vi "Hang Controller.vi"(8 "error in":errorcluster) -> ()   [LabVIEW 2019]
doc: "This VI executes continuously carrying out the current operation and responding to updates or new operations. It will often contain the timing or control code that is difficult to place directly in TeleOp. This VI generally opens all sensors and motors and isolates the rest of the robot code from knowing how the operations are carried out."
uses:
  <vilib>/Rock Robotics/WPI/Framework/Completion Status.ctl
  Hang Setpoints.ctl
  Hang Operations.ctl
  <vilib>/Rock Robotics/WPI/Solenoid/WPI_SolenoidValue.ctl
  <vilib>/Rock Robotics/WPI/Solenoid/WPI_SolenoidChannel.ctl
  <vilib>/Rock Robotics/WPI/ThirdParty/Phoenix-LabVIEW/Motor Controller/Controls/CTRE_Phoenix_MotorControl_ControlMode.ctl
  <vilib>/Rock Robotics/WPI/Solenoid/WPI_SolenoidOpenDouble.vi
  <vilib>/Rock Robotics/WPI/Solenoid/WPI_SolenoidSetEnum.vi
panel:
  in  "Interactive Values":T1
  out "Current\nCmd":string
  in  "Buttons":cluster{"Execute Cmd":bool, "Abort Cmd":bool}
  out "Command Timing":cluster{"Start Time (ms)":u32, "Iterations":i32}
  out "Status":T4
  # "Tip: It may be helpful to observe inputs and sensor values.\nYou may also want to display tuning or debugging controls."
  # "Interactive Command: You may fill in the settings for a command\nand schedule it with the Execute button. You can observe and abort\nany command while fine tuning the code for the controller."
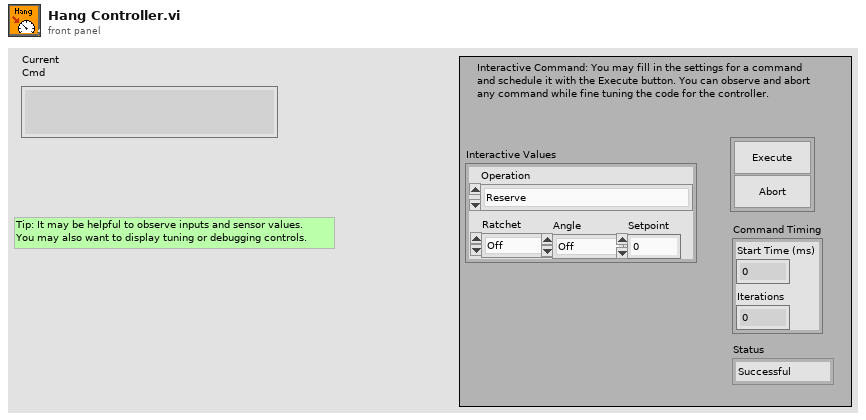
[diagram p1: front panel]
types:
  T1 = typedef "Hang Setpoints.ctl" = cluster{"Operation":T2, "Ratchet":T3, "Angle":T3, "Setpoint":dbl}
  T2 = typedef "Hang Operations.ctl" = enum16{"Reserve", "Read Current", "Immediate"}
  T3 = typedef "WPI_SolenoidValue.ctl" = enum16{"Off", "On", "Forward", "Reverse"}
  T4 = typedef "Completion Status.ctl" = enum16{"Successful", "Aborted", "Incomplete"}
  T5 = typedef "WPI_SolenoidChannel.ctl" = enum8{"Solenoid 0", "Solenoid 1", "Solenoid 2", "Solenoid 3", "Solenoid 4", "Solenoid 5", "Solenoid 6", "Solenoid 7", "Invalid"}
  T6 = typedef "WPI_MotorControlDeviceRef.ctl" = cluster{"DeviceStatus":errorcluster, "Type":T7, "PWM":cluster{"PWM Channel":T8, "DeadBand":T9}, "CAN":cluster{"Device Number":u8, "SetOutput VI Ref":variant, "GetOutput VI Ref":variant, "Enable VI Ref":variant, "Disable VI Ref":variant, "Data":variant}, "Invert":bool, "DIO PWM":cluster{"PWM \"Enable\" Channel":T8, "DIOChannel":T10, "PWM Rate":dbl}}
  T7 = typedef "WPI_MotorControlType.ctl" = enum16{"PWM", "CAN", "DIO PWM"}
  T8 = typedef "FPGA_DIOPWMChannel.ctl" = enum8{"PWM 0", "PWM 1", "PWM 2", "PWM 3", "PWM 4", "PWM 5", "PWM 6", "PWM 7", "PWM 8", "PWM 9", "PWM MXP 0", "PWM MXP 1", "PWM MXP 2", "PWM MXP 3", "PWM MXP 4", "PWM MXP 5", "PWM MXP 6", "PWM MXP 7", "PWM MXP 8", "PWM MXP 9", "Invalid"}
  T9 = typedef "WPI_PWMDeadband.ctl" = cluster{"Name":string, "maxPositivePwm":i32, "minPositivePwm":i32, "centerPwm":i32, "maxNegativePwm":i32, "minNegativePwm":i32, "angularRange":u16}
  T10 = typedef "FPGA_DIOChannel.ctl" = enum8{"DIO 0", "DIO 1", "DIO 2", "DIO 3", "DIO 4", "DIO 5", "DIO 6", "DIO 7", "DIO 8", "DIO 9", "DIO MXP 0", "DIO MXP 1", "DIO MXP 2", "DIO MXP 3", "DIO MXP 4", "DIO MXP 5", "DIO MXP 6", "DIO MXP 7", "DIO MXP 8", "DIO MXP 9", "DIO MXP 10", "DIO MXP 11", "DIO MXP 12", "DIO MXP 13", "DIO MXP 14", "DIO MXP 15", "SPI Port CS1", "SPI Port CS2", "SPI Port CS3", "SPI Port MISO", "SPI Port MOSI", "Invalid"}
  T11 = typedef "WPI_SolenoidDevRef.ctl" = cluster{"DevStatus":errorcluster, "Pneumatics Control Module":u8, "Forward Solenoid Channel":T5, "Reverse Solenoid Channel":T5}
  T12 = typedef "Command Status Info.ctl" = cluster{"Name":string, "Status":T4, "notifier out":T13}
  T13 = typedef "Completion Notifier.ctl" = refnum<notifier>
  T14 = cluster{"Current Command":T1, "Command Timing":cluster{"Start Time (ms)":u32, "Iterations":i32}, "Command Arguments":cluster{"Command Info":T12, "Description":string, "Default Command":T1, "queue out":refnum<queue>, "Subsystem Name":string}}
  T15 = typedef "CTRE_Phoenix_MotorControl_ControlMode.ctl" = u16
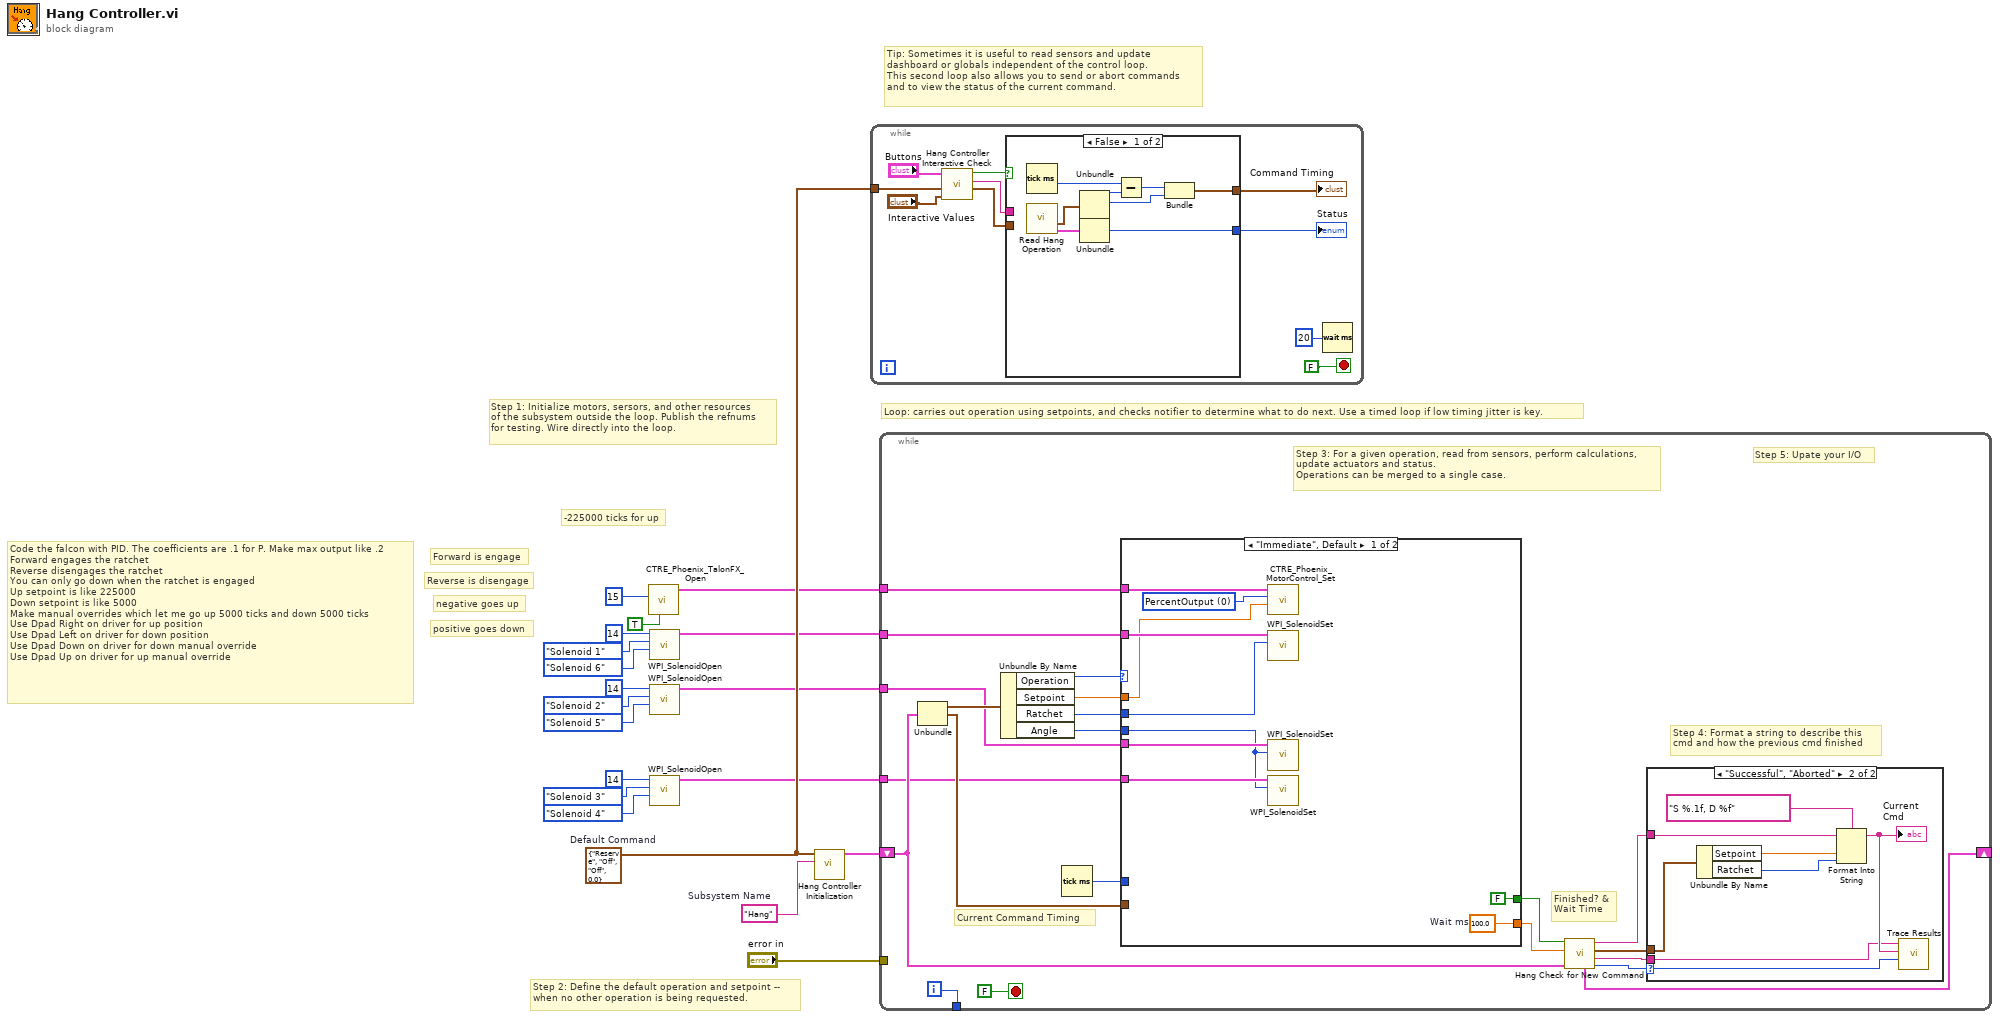
[diagram p0: block diagram]
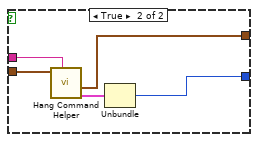
[diagram p2: hidden frame]
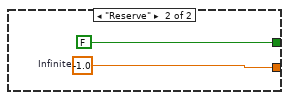
[diagram p3: hidden frame]
diagram:
  w16 = T1 {"Operation"=enum."Reserve", "Ratchet"=enum."Off", "Angle"=enum."Off", "Setpoint"=0.0}  # Default Command
  w17 = "Hang"  # Subsystem Name
  # "Code the falcon with PID. The coefficients are .1 for P. Make max output like .2\nForward engages the ratchet\nReverse disengages the ratchet\nYou can only go down when the ratchet is engaged\nUp setpoint is like 225000\nDown setpoint is like 5000\nMake manual overrides which let me go up 5000 ticks and down 5000 ticks\nUse Dpad Right on driver for up position\nUse Dpad Left on driver for down position\nUse Dpad Down on driver for down manual override\nUse Dpad Up on driver for up manual override"
  # "-225000 ticks for up"
  # "positive goes down"
  # "negative goes up"
  # "Reverse is disengage"
  # "Forward is engage"
  # "Tip: Sometimes it is useful to read sensors and update\ndashboard or globals independent of the control loop.\nThis second loop also allows you to send or abort commands\nand to view the status of the current command."
  # "Step 2: Define the default operation and setpoint --\nwhen no other operation is being requested."
  # "Step 1: Initialize motors, sersors, and other resources\nof the subsystem outside the loop. Publish the refnums\nfor testing. Wire directly into the loop."
  # "Loop: carries out operation using setpoints, and checks notifier to determine what to do next. Use a timed loop if low timing jitter is key."
  n1 = call <vilib>:"CTRE_Phoenix_TalonFX_Open.vi"("Invert"=TRUE, "Device Number"=u8 15) -> ("CAN Talon SRX Ref"=w7:T6)  [unwired: 8 in, 1 out]
  n2 = call-poly <vilib>:"WPI_SolenoidOpen.vi"("Reverse Solenoid Channel"=WPI_SolenoidChannel."Solenoid 6", "Forward Solenoid Channel"=WPI_SolenoidChannel."Solenoid 1", "Pneumatics Control Module (0)"=u8 14) -> ("SolenoidDevRef"=w11:T11)  [unwired: 7 in, 1 out]
  n3 = call-poly <vilib>:"WPI_SolenoidOpen.vi"("Reverse Solenoid Channel"=WPI_SolenoidChannel."Solenoid 5", "Forward Solenoid Channel"=WPI_SolenoidChannel."Solenoid 2", "Pneumatics Control Module (0)"=u8 14) -> ("SolenoidDevRef"=w12:T11)  [unwired: 7 in, 1 out]
  n4 = call-poly <vilib>:"WPI_SolenoidOpen.vi"("Reverse Solenoid Channel"=WPI_SolenoidChannel."Solenoid 4", "Forward Solenoid Channel"=WPI_SolenoidChannel."Solenoid 3", "Pneumatics Control Module (0)"=u8 14) -> ("SolenoidDevRef"=w14:T11)  [unwired: 7 in, 1 out]
  n5 = call "Hang Controller Initialization.vi"("Subsystem Name"=w17, "Default Command"=w16) -> ("Current Command"=w18:T14)  [unwired: 9 in]
  n6 = while {
    tunnel: w16 -> [w26]
    stop <- FALSE stop-if-true
    n7 = call "Hang Controller Interactive Check.vi"("Interactive Command in"="Interactive Values", "Default Command"=w26, "Buttons"="Buttons") -> ("Interactive Command out"=w23:T1, "Trace String"=w24:string, "Schedule"=w25:bool)  [unwired: 6 in]
    n8 = case shown="False" w25 {
      tunnel: [w37 w42] -> w22
      tunnel: w23 -> [_ w40]
      tunnel: [w33 w38] -> w21
      tunnel: w24 -> [_ w41]
      frame False {
        n9 = Tick Count (ms)() -> (millisecond timer value=w32:u32)
        n10 = call "Read Hang Operation.vi"() -> ("Command Info"=w30:T12, "SubSystem Data"=w31:T1)  [unwired: 9 in, 1 out]
        n11 = Unbundle(w31) -> ("Operation"=w36:T2, "Ratchet"=w34:T3)  [unwired: 2 out]
        n12 = Unbundle(w30) -> ("Status"=w37:T4)  [unwired: 2 out]
        n13 = Subtract(x=w32, y=w36) -> (x-y=w35:u32)
        n14 = Bundle(w35, "Ratchet"=w34) -> (w33:cluster{u32, "Ratchet":T3})  [unwired: 1 in]
      }
      frame True {
        n15 = call "Hang Command Helper.vi"("Description"=w41, "SubSystem Data"=w40) -> ("Command Info Out"=w39:T12, "Command Timing"=w38:cluster{"Start Time (ms)":u32, "Iterations":i32})  [unwired: 7 in, 1 out]
        n16 = Unbundle(w39) -> ("Status"=w42:T4)  [unwired: 2 out]
      }
    }
    "Status" <- w22
    "Command Timing" <- w21
    n17 = Wait (ms)(milliseconds to wait=u32 20) -> ()  [unwired: 1 out]
  }
  n18 = while {
    shift-right: [w56] -> _
    shift-left: w18 -> [w49]
    tunnel: [w62] -> _
    tunnel: "error in" -> [_]
    tunnel: w14 -> [w46]
    tunnel: w12 -> [w45]
    tunnel: w11 -> [w48]
    tunnel: w7 -> [w43]
    i -> [w62]
    stop <- FALSE stop-if-true
    # "Step 5: Upate your I/O"
    # "Step 4: Format a string to describe this\ncmd and how the previous cmd finished"
    # "Current Command Timing"
    # "Finished? &\nWait Time"
    # "Step 3: For a given operation, read from sensors, perform calculations,\nupdate actuators and status.\nOperations can be merged to a single case."
    n19 = Unbundle(w49) -> ("Current Command"=w61:T1, "Command Timing"=w58:cluster{"Start Time (ms)":u32, "Iterations":i32})  [unwired: 1 out]
    n20 = Unbundle By Name(w61) -> ("Operation"=w60:T2, "Setpoint"=w44:dbl, "Ratchet"=w57:T3, "Angle"=w47:T3)
    n21 = Tick Count (ms)() -> (millisecond timer value=w59:u32)
    n22 = case shown="\"Immediate\", Default" w60 {
      tunnel: [w73 w75] -> w54
      tunnel: [FALSE ("ignore previous (F)") FALSE ("ignore previous (F)")] -> w55
      tunnel: w58 -> [_ _]
      tunnel: w59 -> [_ _]
      tunnel: w57 -> [w64 _]
      tunnel: w43 -> [w72 _]
      tunnel: w45 -> [w70 _]
      tunnel: w46 -> [w69 _]
      tunnel: w48 -> [w68 _]
      tunnel: w47 -> [w66 _]
      tunnel: w44 -> [w65 _]
      frame "Immediate", Default {
        w71 = T15 0 items=["PercentOutput"=0, "Position"=1, "Velocity"=2, "Current"=3, "Follower"=5, "MotionProfile"=6, "MotionMagic"=7, "MotionProfileArc"=10, "Disabled"=15] ("Control Mode")
        w73 = 100.0  # Wait ms
        n23 = call <vilib>:"CTRE_Phoenix_MotorControl_Set.vi"("Output"=w65, "Control Mode"=w71, "PhoenixMotorControlDevRef"=w72) -> ()  [unwired: 7 in, 2 out]
        n24 = call-poly <vilib>:"WPI_SolenoidSet.vi"("Value"=w64, "SolenoidDevRef"=w68) -> ()  [unwired: 8 in, 2 out]
        n25 = call-poly <vilib>:"WPI_SolenoidSet.vi"("Value"=w66, "SolenoidDevRef"=w70) -> ()  [unwired: 8 in, 2 out]
        n26 = call-poly <vilib>:"WPI_SolenoidSet.vi"("Value"=w66, "SolenoidDevRef"=w69) -> ()  [unwired: 8 in, 2 out]
      }
      frame "Reserve" {
        w75 = -1.0  # Infinite
      }
    }
    n27 = call "Hang Check for New Command.vi"("Current Command"=w49, "Wait time (ms)"=w54, "Finished?"=w55) -> ("Completion"=w50:T4, "Subsystem Name"=w51:string, "Current Command"=w52:T1, "Initial Trace String"=w53:string, "NextCommand"=w56:T14)  [unwired: 4 in]
    n28 = case shown="\"Successful\", \"Aborted\"" w50 {
      selector: w50 -> [_ w83]
      tunnel: w53 -> [_ w79]
      tunnel: w52 -> [_ w80]
      tunnel: w51 -> [_ w76]
      frame "Incomplete", Default {
        # "Continuing current command"
      }
      frame "Successful", "Aborted" {
        # "Report and setup for next command"
        n29 = Unbundle By Name(w80) -> ("Setpoint"=w82:dbl, "Ratchet"=w77:T3)
        n30 = Format Into String(format string="S %.1f, D %f", initial string=w79, w82, w77) -> (resulting string=w78:string)  [unwired: 1 in, 1 out]
        "Current\nCmd" <- w78
        n31 = call <vilib>:"Trace Results.vi"("Status of previous command"=w83, "Description"=w78, "Subsystem"=w76) -> ()  [unwired: 9 in]
      }
    }
  }
